vi "Release ActorRef Queue.vi"(8 "error in (no error)":errorcluster, 11 "Core In":refnum<class "Core.lvclass">) -> (0 "error out":errorcluster, 3 "Core Out":refnum<class "Core.lvclass">)   [LabVIEW 2019, in "Core.lvlib" / "Core.lvclass"]
uses:
  Core.lvclass
  ModuleAbstract/ModuleAbstract.lvclass
  C:/Projekty/_Wewnetrzne/PC_ActorFramework/07_Program/LABVIEW/02_Source/Modules/ModuleAbstract/ModuleAbstract.lvclass
  C:/Program Files (x86)/National Instruments/LabVIEW 2019/vi.lib/ActorFramework/Actor/Actor.lvclass
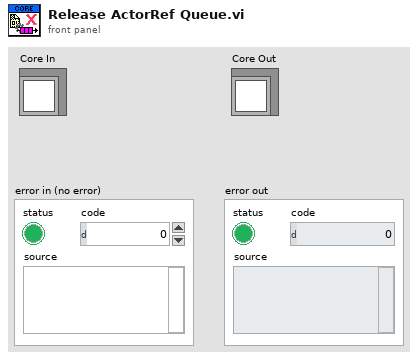
[diagram p1: front panel]
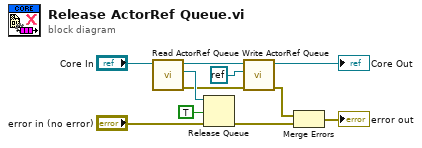
[diagram p0: block diagram]
diagram:
  n1 = call "Read ActorRef Queue.vi"("ModuleAbstract in"="Core In") -> ("error out"=w3:errorcluster, "ActorRef Queue"=w7:refnum<queue>, "ModuleAbstract out"=w8:refnum<class "Core.lvclass">)  [unwired: 8 in]
  n2 = Release Queue(queue=w7, force destroy? (F)=TRUE, error in (no error)="error in (no error)") -> (error out=w6:errorcluster)  [unwired: 2 out]
  n3 = call "Write ActorRef Queue.vi"("error in (no error)"=w3, "ActorRef Queue"=refnum<k0> refnum, "ModuleAbstract in"=w8) -> ("error out"=w1:errorcluster, "ModuleAbstract out"=→"Core Out":refnum<class "Core.lvclass">)  [unwired: 7 in]
  n4 = Merge Errors(w1, w6) -> (→"error out":errorcluster)
